vi "Fetch Waveform.vi"(8 "error in (no error)":errorcluster, 10 "Channel (1)":i32(ring)=1 items=["1"=1, "2"=2, "3"=3, "4"=4], 11 "VISA resource name":refnum<visa-resource-name>) -> (0 "error out":errorcluster, 2 "Waveform Array":dbl[](array[numeric]) format="%^.3e", 3 "VISA resource name out":refnum<visa-resource-name>, 4 "Initial X":dbl format="%^.3e", 5 "X Increment":dbl format="%^.3e")   [LabVIEW 2020, in "Rohde&Schwarz RTx Oscilloscopes.lvlib"]
doc: "This function returns the waveform the oscilloscope acquires for the channel you specify. The waveform is from an acquisition that you previously initiated.\n\nYou use the Initiate Acquisition.vi to start an acquisition on the channels that you enable with the Configure Channel.vi. The oscilloscope acquires waveforms for the enabled channels concurrently. You must call this function separately for each enabled channel to obtain the waveforms.\n\nYou can call the Read Waveform.vi instead of the Initiate Acquisition.vi. The Read Waveform.vi starts an acquisition on all enabled channels, waits for the acquisition to complete, and returns the waveform for the channel you specify. You call this function to obtain the waveforms for each of the remaining channels.\n\nNotes:\n- After this function executes, each element in the Waveform Array parameter is either a voltage or a value indicating that the oscilloscope could not sample a voltage.\n- You configure the interpolation method the oscilloscope uses with the Configure Interpolation.vi. If you disable interpolation, the oscilloscope does not interpolate points in the waveform.\n- This function does not check the instrument status. Typically, you call this function only in a sequence of calls to other low-level driver functions. The sequence performs one operation. You use the low-level functions to optimize one or more aspects of interaction with the instrument. If you want to check the instrument status, call the Error Query.vi at the conclusion of the sequence.\n\nAttributes:\nRSRTX_ATTR_WAVEFORM_CONVERSION_X_START\nRSRTX_ATTR_WAVEFORM_CONVERSION_X_INCREMENT\n\nRemote-control commands:\nFORMat REAL,32\nCHANnel<m>[:WAVeform<n>]:DATA[:VALues]"
uses:
  Rohde&Schwarz RTx Oscilloscopes.lvlib
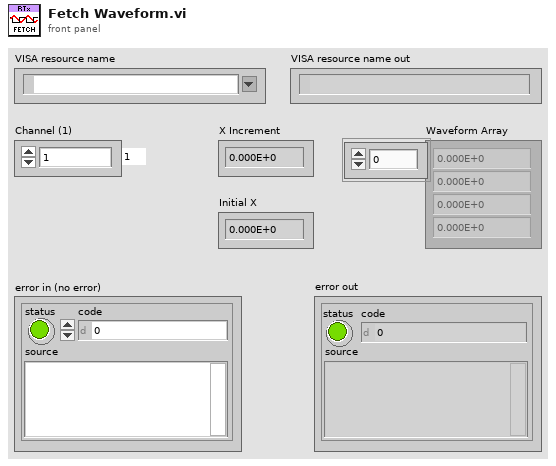
[diagram p1: front panel]
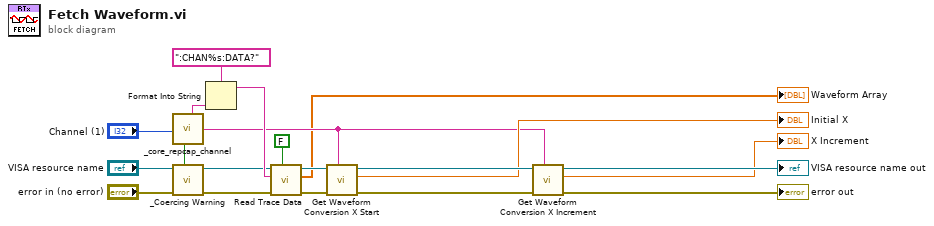
[diagram p0: block diagram]
diagram:
  n1 = call "_core_repcap_channel.vi"("Channel In"="Channel (1)") -> ("In Range?"=w4:bool, "Channel cmdValue Out"=w3:string, "Channel Identifier Out"=w2:string)
  n2 = call "_Coercing Warning.vi"("In Range?"=w4, "error in"="error in (no error)", "VISA resource name"="VISA resource name") -> ("error out"=w16:errorcluster, "VISA resource name out"=w15:refnum<visa-resource-name>)  [unwired: 7 in]
  n3 = Format Into String(format string=":CHAN%s:DATA?", w3) -> (resulting string=w19:string)  [unwired: 2 in, 1 out]
  n4 = call "Read Trace Data.vi"("Wait for OPC (F)"=FALSE, "error in"=w16, "Query"=w19, "VISA session"=w15) -> ("error out"=w14:errorcluster, "Trace Data"=→"Waveform Array":dbl[], "dup VISA session"=w13:refnum<visa-resource-name>)  [unwired: 4 in, 1 out]
  n5 = call "Get Waveform Conversion X Start"("Repeated Capabilities"=w2, "error in (no error)"=w14, "instrument handle"=w13) -> ("error out"=w12:errorcluster, "Waveform Conversion X Start"=→"Initial X":dbl, "instrument handle out"=w11:refnum<visa-resource-name>)  [unwired: 6 in]
  n6 = call "Get Waveform Conversion X Increment"("Repeated Capabilities"=w2, "error in (no error)"=w12, "instrument handle"=w11) -> ("error out"=→"error out":errorcluster, "Waveform Conversion X Increment"=→"X Increment":dbl, "instrument handle out"=→"VISA resource name out":refnum<visa-resource-name>)  [unwired: 6 in]
